vi "main.vi"() -> ()   [LabVIEW 2014]
uses:
  <vilib>/addons/Sound and Vibration/svt_Controls/subVIs/Multiplot Octave Graph.ctl
  <vilib>/Utility/NIReport.llb/NI_report.lvclass
  <vilib>/Utility/NIReport.llb/HTML Report Image Alignment.ctl
  <vilib>/sound2/lvsound2.llb/Sound File Read Open.vi
  <vilib>/sound2/lvsound2.llb/Sound File Info (refnum).vi
  <vilib>/sound2/lvsound2.llb/Sound File Read (DBL).vi
  <vilib>/addons/Sound and Vibration/svt_Octave/SVT Third-octave Analysis (1 Ch).vi
  <vilib>/addons/Sound and Vibration/svt_Octave/SVT Octave Analysis (1 Ch).vi
  <vilib>/measure/matone.llb/Harmonic Distortion Analyzer 1 Chan.vi
  <vilib>/addons/Sound and Vibration/svt_Transients/SVT STFT vs Time (Intensity).vi
  <vilib>/printing/ReportDocExtensions.llb/Append Front Panel Image to Report (path).vi
  <vilib>/addons/Sound and Vibration/svt_Octave/SoundVib_Octave.lvlib
  <vilib>/Analysis/NI_AALPro.lvlib
  <vilib>/measure/NI_MAPro.lvlib
  <vilib>/addons/Sound and Vibration/svt_Transients/SoundVib_Transient.lvlib
  <vilib>/Utility/NIReport.llb/Excel/NI_Excel.lvclass
  <vilib>/Utility/NIReport.llb/NI_ReportGenerationCore.lvlib
panel:
  in  "Print Button":bool
  in  "Help Button":bool
  in  "Tab Control":T1(tab)
  out "Wave":dbl[][](graph)
  in  "Play":bool
  in  "Pa / dBA":bool
  out "Multiplot":T2
  in  "Octave":bool
  in  "Тип анализа":u16(ring)=1 items=["1/3 октавный", "Октавный"]
  in  "Режим усреднения":u16(ring)=1 items=["Linear", "Exponential", "Equal confidence", "Peak"]
  out "Эталон":T3 {"band power" format="%#.2g"}
  out "Разность":T3 {"band power" format="%#.2g"}
  out "FFT 2":dbl[][](graph)
  out "Ампл. спектр (от. ед.)":dbl[][](array[numeric])
  out "THD (%)":dbl[](array[numeric])
  in  "FFT":bool
  in  "Режим экспорта THD":T4(ring)
  out "STFT":dbl[][](graph)
  in  "SFFT":bool
  in  "Тип оконной обработки":T5(ring)=enum."Hanning"
  in  "Время анализа (%)":dbl=50.0 min=1.0 max=100.0 step=1.0
  in  "Тип отображения":T6(ring)=enum."rainbow"
  out "Selected":i32
  in  "Обрабатываемый файл":string(combo)
  out "Start":i32
  out "Finish":i32
  in  "Clear":bool
  in  "stop":bool
  in  "TypeD":T7=enum."Open Files"
  in  "Open Files":bool
  # "Автоматизированная система объективизации оценки степени совпадения двух сравниваемых электронных звуковых рядов по заданому набору параметров"
  # "Осн. частота (Гц)"
  # "Мощность (дБ)"
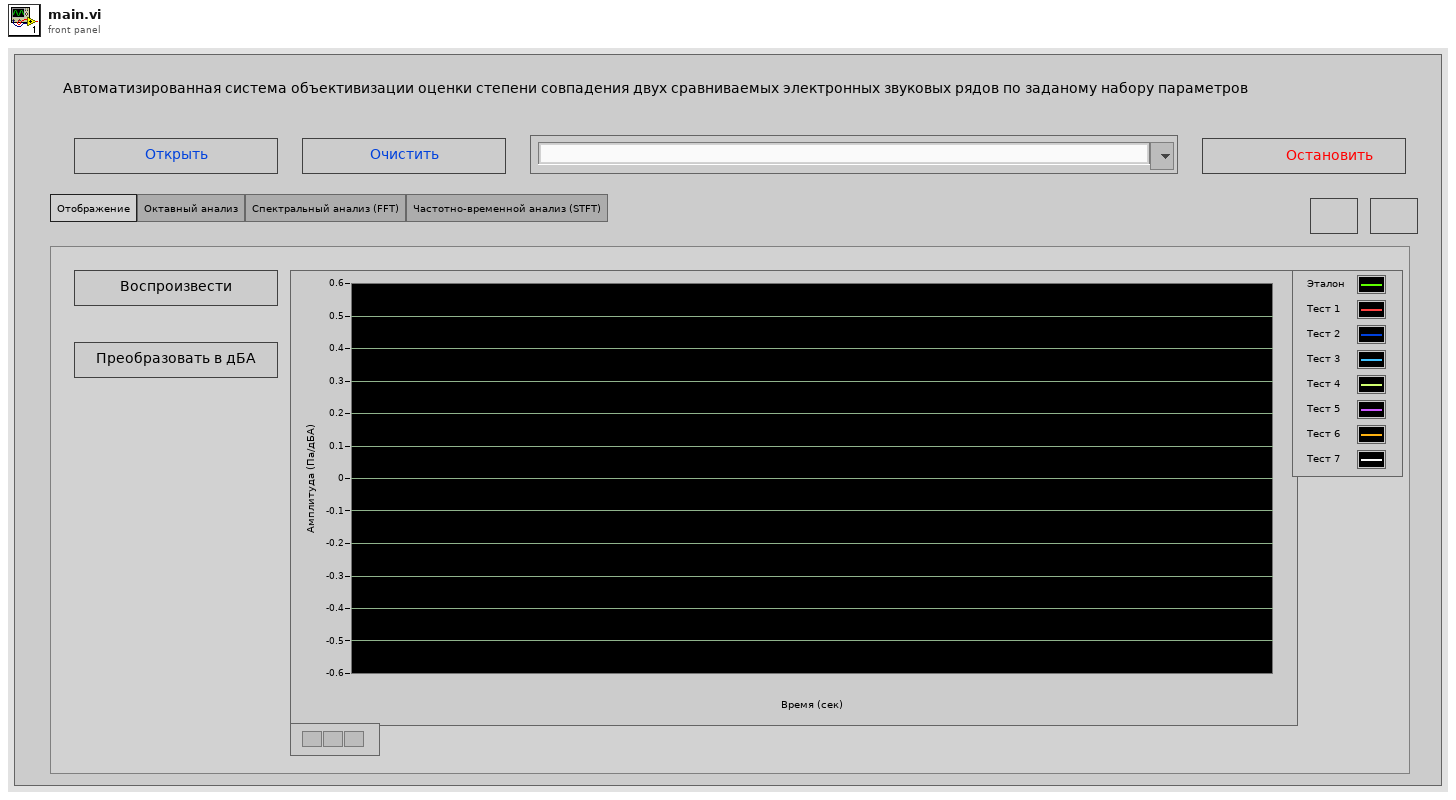
[diagram p1: front panel]
types:
  T1 = enum32{"Отображение", "Октавный анализ", "Спектральный анализ (FFT)", "Частотно-временной анализ (STFT)"}
  T2 = typedef "Multiplot Octave Graph.ctl" = cluster{"nominal frequencies [Hz]":dbl[], "band power [dB EU]":dbl[]}[]
  T3 = cluster{"nominal frequencies [Hz]":dbl[], "band power":dbl[]}
  T4 = enum16{"none", "input signal", "fundamental signal", "residual signal", "harmonics only", "noise and spurs"}
  T5 = enum16{"None ", "Hanning", "Hamming", "Blackman-Harris", "Exact Blackman", "Blackman", "Flat Top", "4 Term B-Harris ", "7 Term B-Harris", "Low Sidelobe"}
  T6 = enum16{"fire", "rainbow", "grey", "inverse grey", "ice", "original"}
  T7 = typedef "TypeDef1.ctl" = enum16{"Initialize", "Idle", "Open Files", "Pa_dBA", "FFT", "SFFT", "Play", "Octave", "Print", "Shutdown"}
  T8 = cluster{"nominal frequencies [Hz]":dbl[], "band power":dbl[]}[]
  T9 = enum16{"open", "open or create", "create or replace", "create", "open (read only)"}
  T10 = cluster{" mode":enum16{"Slow", "Fast", "Impulse", "Custom"}, "time constant [ms]":dbl}
  T11 = cluster{"low band":enum16{"20 Hz", "25 Hz", "31.5 Hz", "40 Hz", "50 Hz", "63 Hz", "80 Hz", "100 Hz", "125 Hz", "160 Hz", "200 Hz", "250 Hz", "315 Hz", "400 Hz", "500 Hz", "630 Hz", "800 Hz", "1000 Hz", "1250 Hz", "1600 Hz", "2000 Hz", "2500 Hz", "3150 Hz", "4000 Hz", "5000 Hz", "6300 Hz", "8000 Hz", "10000 Hz", "12500 Hz", "16000 Hz", "20000 Hz"}, "high band":enum16{"20 Hz", "25 Hz", "31.5 Hz", "40 Hz", "50 Hz", "63 Hz", "80 Hz", "100 Hz", "125 Hz", "160 Hz", "200 Hz", "250 Hz", "315 Hz", "400 Hz", "500 Hz", "630 Hz", "800 Hz", "1000 Hz", "1250 Hz", "1600 Hz", "2000 Hz", "2500 Hz", "3150 Hz", "4000 Hz", "5000 Hz", "6300 Hz", "8000 Hz", "10000 Hz", "12500 Hz", "16000 Hz", "20000 Hz"}}
  T12 = cluster{"low band":enum16{"16 Hz", "31.5 Hz", "63 Hz", "125 Hz", "250 Hz", "500 Hz", "1000 Hz", "2000 Hz", "4000 Hz", "8000 Hz", "16000 Hz"}, "high band":enum16{"16 Hz", "31.5 Hz", "63 Hz", "125 Hz", "250 Hz", "500 Hz", "1000 Hz", "2000 Hz", "4000 Hz", "8000 Hz", "16000 Hz"}}
  T13 = typedef "NI_ReportGenerationCore.lvlib/HTML Report Image Alignment.ctl" = enum16{"(default)", "LEFT", "RIGHT", "TOP", "TEXTTOP", "MIDDLE", "ABSMIDDLE", "BASELINE", "BOTTOM", "ABSBOTTOM"}
  T14 = enum16{"Standard Report", "HTML", "Word", "Excel"}
  T15 = typedef "Sound File Refnum.ctl" = refnum<file>
  T16 = typedef "SoundVib_Octave.lvlib/sv_Octave Info.ctl" = cluster{"standard":enum16{"ANSI S.1.11", "IEC 1260"}, "bandwidth":enum16{"1 octave", "1/3 octave", "1/6 octave", "1/12 octave", "1/24 octave"}, "low band":i32, "high band":i32, "weighting filter":T17, "dB reference":dbl, "dB On":bool, "unit label":string, "channel name":string, "description":string, "engineering units":T18, "custom label":string, "spectrum type":enum16{"power", "magnitude"}, "spectral density":bool, "filters settled":bool}
  T17 = typedef "svc_Weighting Filter Text Ring.ctl" = u16
  T18 = typedef "svc_Engineering Units Text Ring.ctl" = u16
  T19 = cluster{dbl, dbl, "Время анализа (%)":dbl, "time increment units (%)":enum16{"%", "s", "ms"}}
  T20 = enum32{"invalid app kind", "Development System", "Run Time System", "Student Edition", "Embedded LabVIEW", "Evaluation", "Custom"}
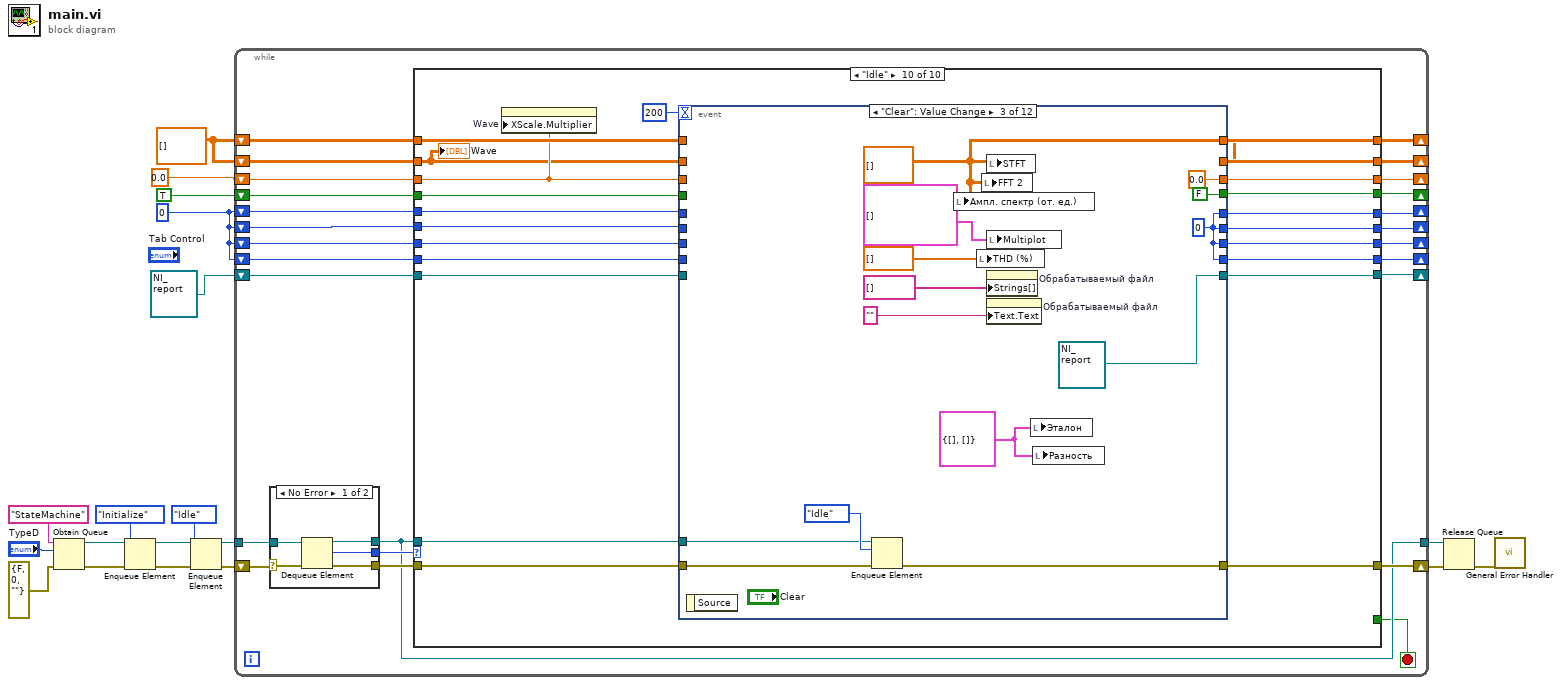
[diagram p0: block diagram]
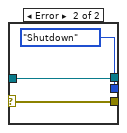
[diagram p2: hidden frame]
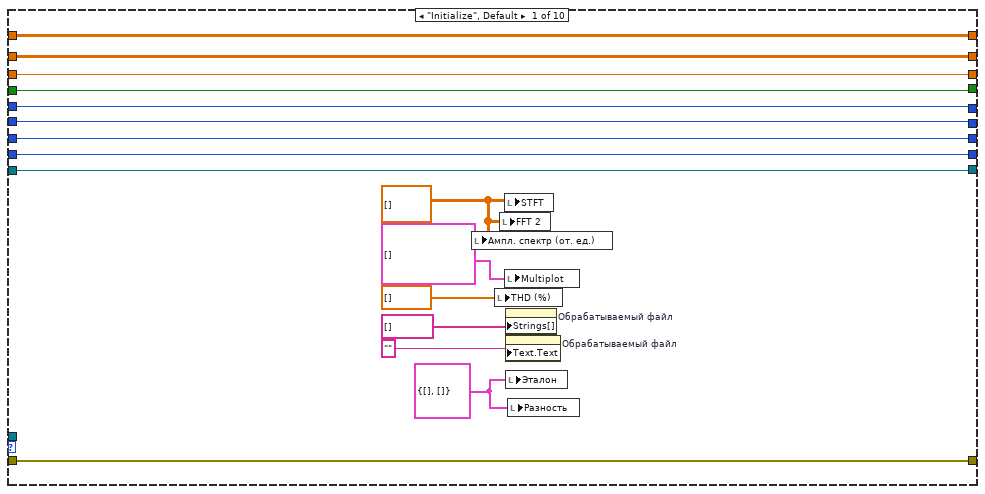
[diagram p3: hidden frame]
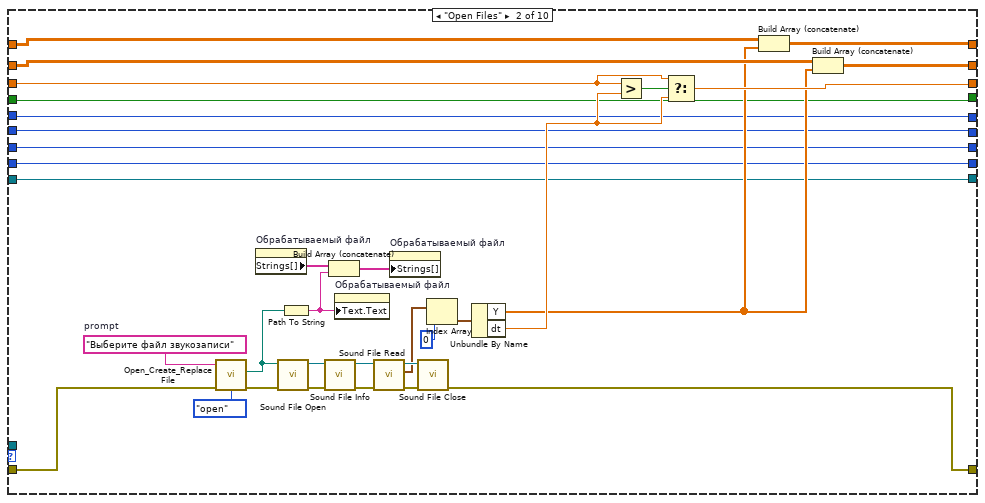
[diagram p4: hidden frame]
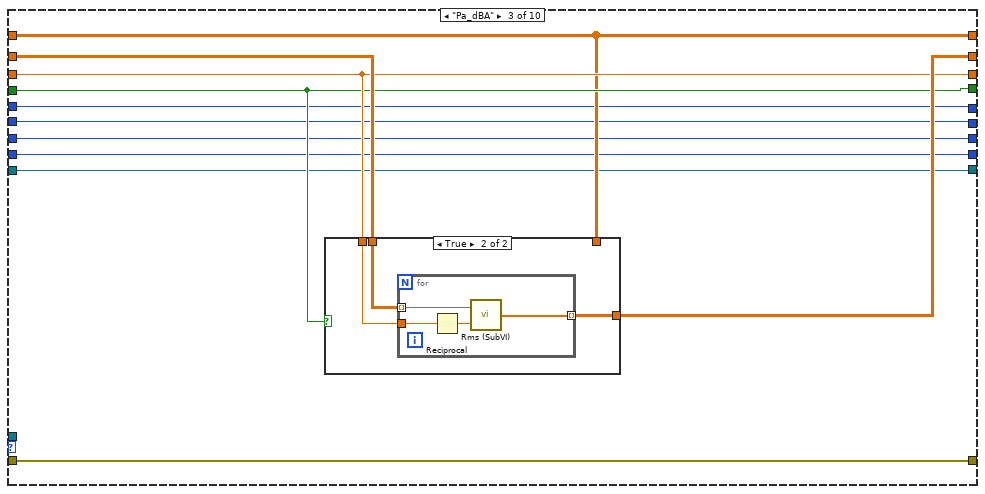
[diagram p5: hidden frame]
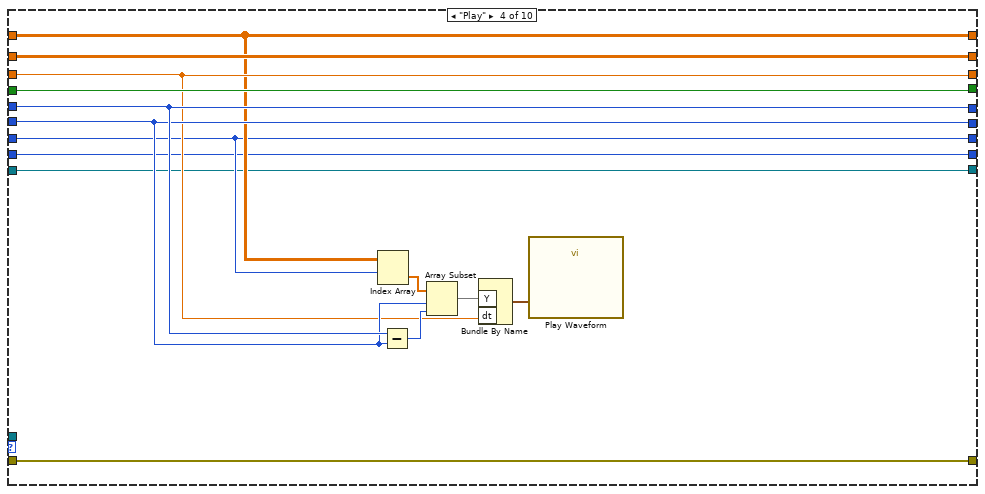
[diagram p7: hidden frame]
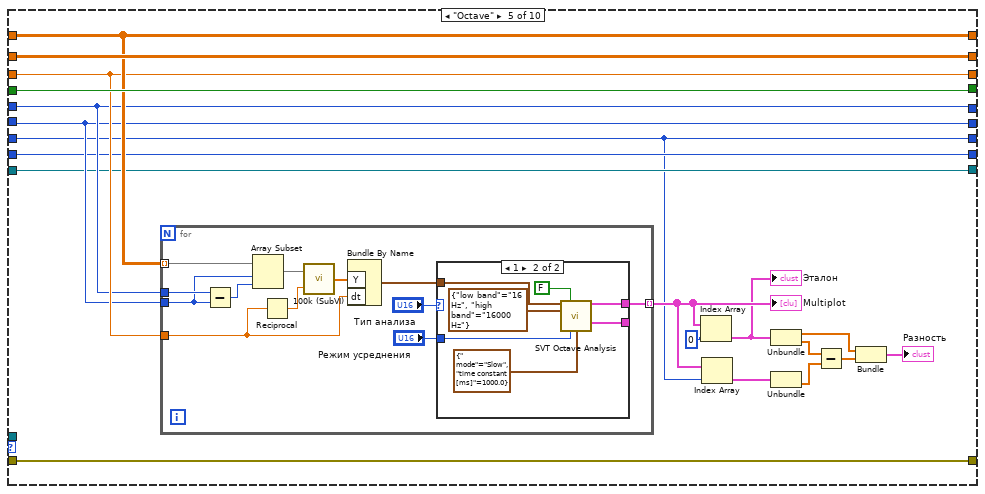
[diagram p8: hidden frame]
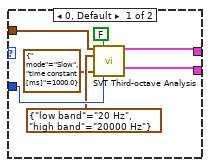
[diagram p9: hidden frame]
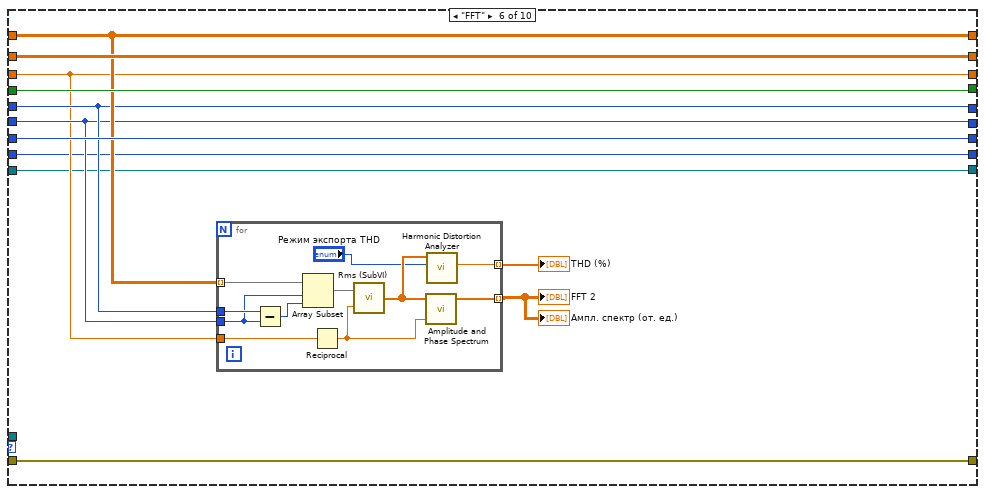
[diagram p10: hidden frame]
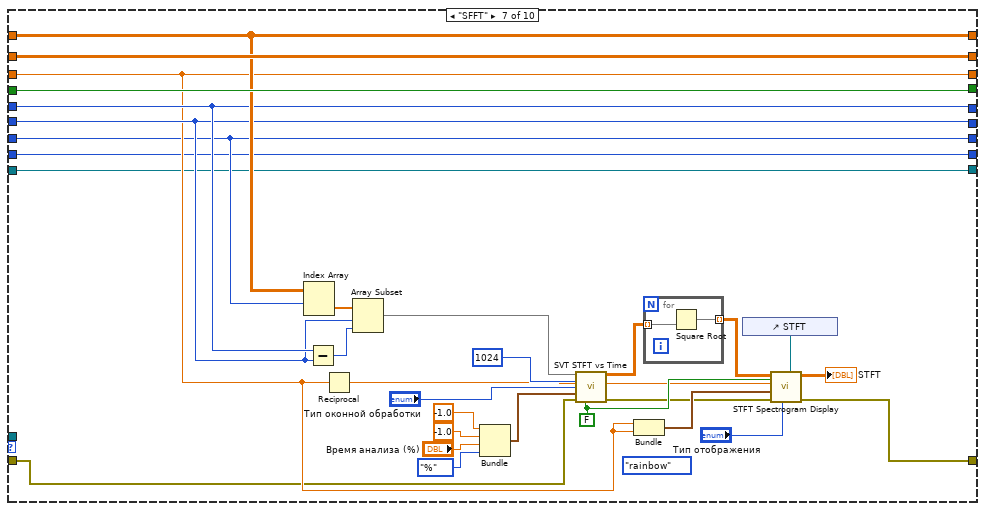
[diagram p11: hidden frame]
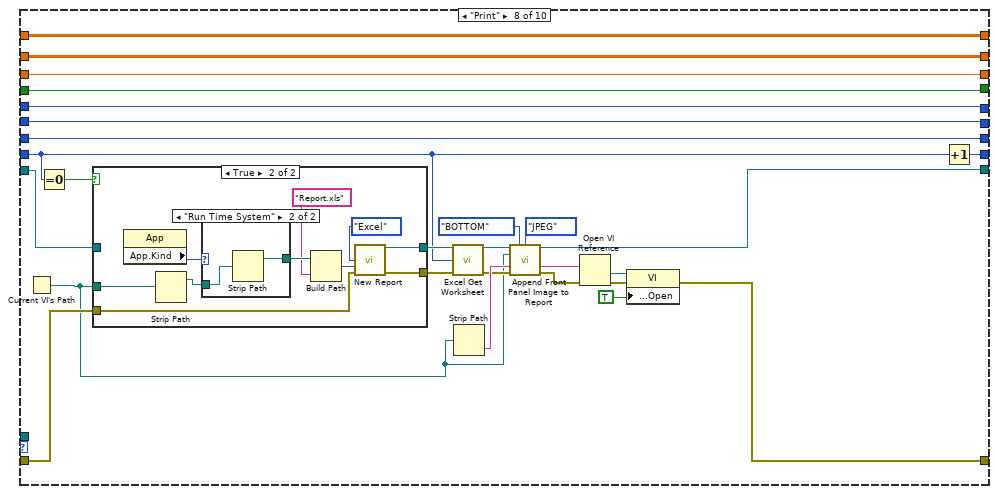
[diagram p12: hidden frame]
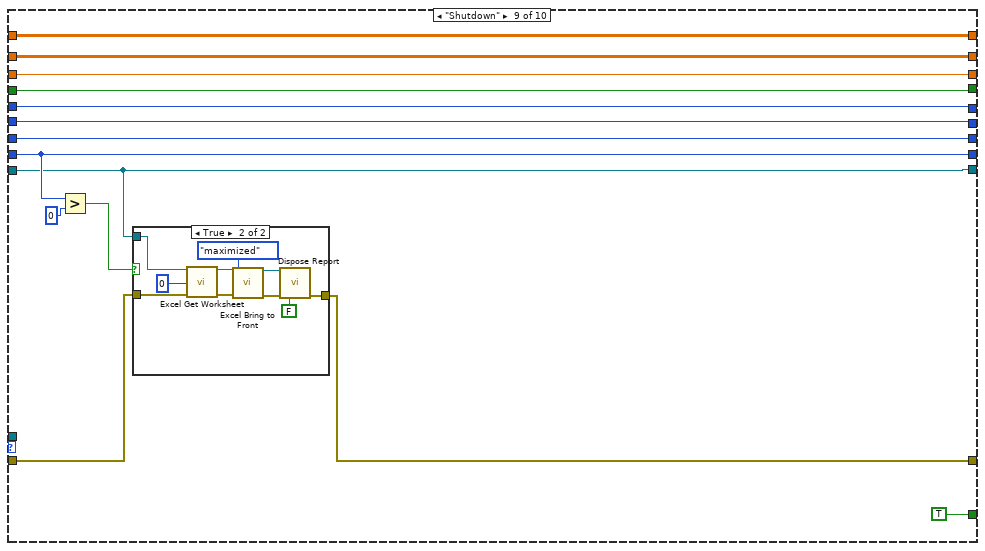
[diagram p15: hidden frame]
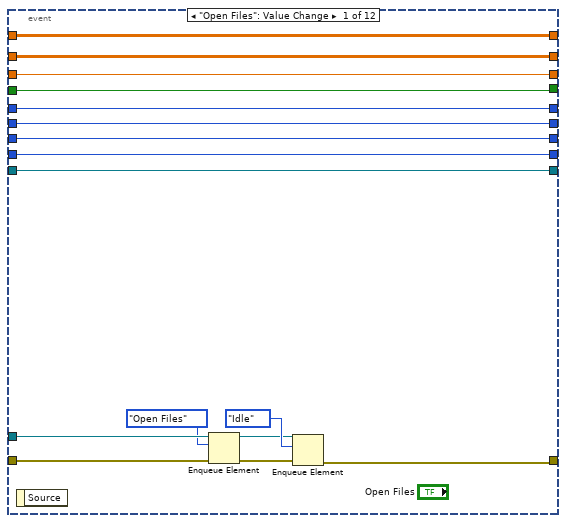
[diagram p17: hidden frame]
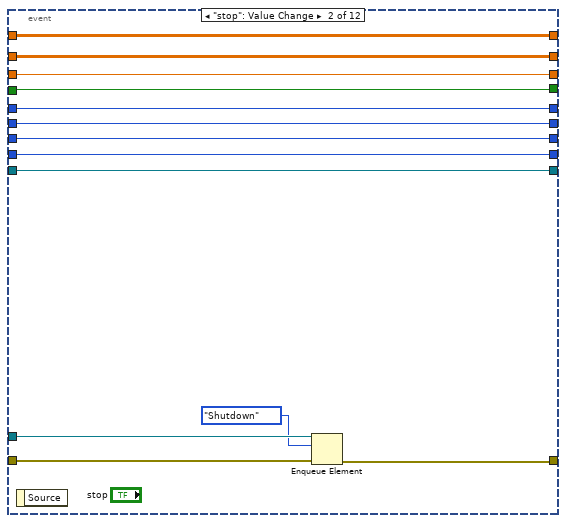
[diagram p18: hidden frame]
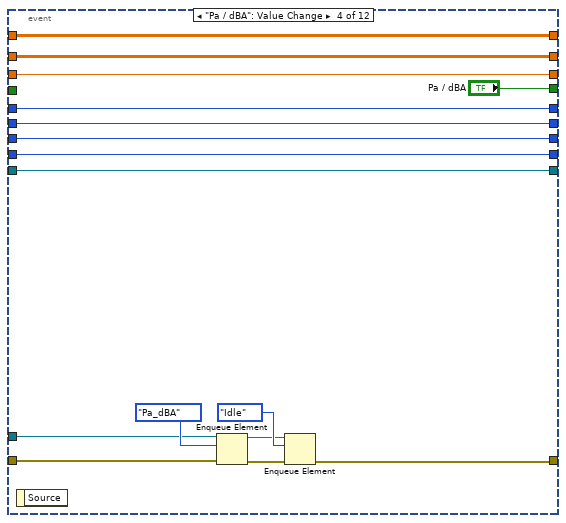
[diagram p19: hidden frame]
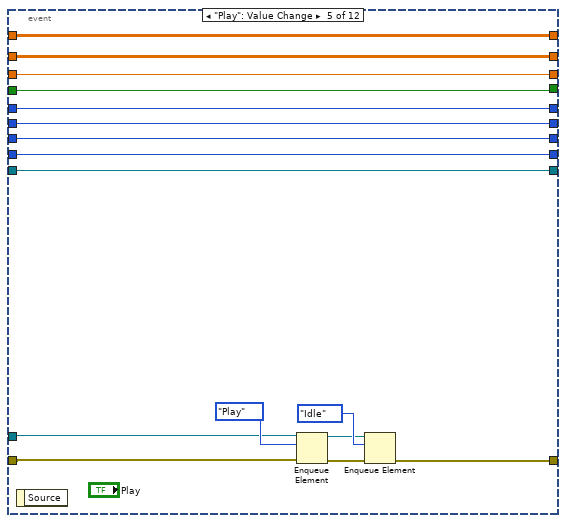
[diagram p20: hidden frame]
diagram:
  w3 = 0
  w9 = dbl[][] []
  n1 = Obtain Queue(name (unnamed)="StateMachine", element data type="TypeD", error in (no error)=errorcluster {"status"=FALSE, "code"=0, "source"=""}) -> (queue out=w19:refnum<queue>, error out=w18:errorcluster)  [unwired: 2 in, 1 out]
  n2 = Enqueue Element(queue=w19, element=TypeDef1."Initialize", error in (no error)=w18) -> (queue out=w7:refnum<queue>, error out=w6:errorcluster)  [unwired: 1 in, 1 out]
  n3 = Enqueue Element(queue=w7, element=TypeDef1."Idle", error in (no error)=w6) -> (queue out=w4:refnum<queue>, error out=w5:errorcluster)  [unwired: 1 in, 1 out]
  n4 = while {
    tunnel: w4 -> [w43]
    shift-right: [w40] -> w13
    shift-left: w5 -> [w44]
    tunnel: [w39] -> w12
    shift-right: [w36] -> _
    shift-left: w9 -> [w37]
    shift-right: [w35] -> _
    shift-left: 0.0 -> [w24]
    shift-right: [w33] -> _
    shift-left: TRUE -> [w34]
    shift-right: [w31] -> _
    shift-left: w9 -> [w32]
    shift-right: [w28] -> _
    shift-left: w3 -> [w30]
    shift-right: [w27] -> _
    shift-left: w3 -> [w29]
    shift-right: [w25] -> _
    shift-left: w3 -> [w26]
    shift-right: [w22] -> _
    shift-left: w3 -> [w23]
    shift-right: [w20] -> _
    shift-left: refnum<class "NI_report.lvclass"> refnum ("report in") -> [w21]
    stop <- w38 stop-if-true
    n5 = case shown="No Error" w44 {
      selector: w44 -> [w49 w51]
      tunnel: w43 -> [w48 w52]
      tunnel: [w47 w52] -> w39
      tunnel: [w46 w51] -> w41
      tunnel: [w45 TypeDef1."Shutdown"] -> w42
      frame No Error {
        n6 = Dequeue Element(queue=w48, error in (no error)=w49) -> (queue out=w47:refnum<queue>, element=w45:T7, error out=w46:errorcluster)  [unwired: 1 in, 1 out]
      }
      frame Error {
      }
    }
    n7 = case shown="\"Idle\"" w42 {
      tunnel: w41 -> [w68 w72 w112 w124 w151 w184 w211 w251 w278 w322]
      tunnel: [w68 w88 w112 w124 w151 w184 w215 w236 w277 w321] -> w40
      tunnel: w39 -> [_ _ _ _ _ _ _ _ _ w320]
      tunnel: [_ _ _ _ _ _ _ _ TRUE _] -> w38
      tunnel: w37 -> [w67 w89 w111 w126 w152 w191 w232 w259 w288 w310]
      tunnel: [w67 w90 w110 w126 w152 w191 w232 w259 w288 w319] -> w36
      tunnel: [w66 w84 w109 w127 w149 w185 w219 w258 w287 w318] -> w35
      tunnel: w24 -> [w66 w86 w109 w127 w149 w185 w219 w258 w287 w313]
      tunnel: w34 -> [w65 w77 w108 w130 w153 w190 w231 w257 w285 w317]
      tunnel: [w65 w77 w108 w130 w153 w190 w231 w257 w285 w316] -> w33
      tunnel: w32 -> [w64 w83 w107 w125 w150 w188 w222 w260 w286 w315]
      tunnel: [w64 w81 w107 w125 w150 w188 w222 w260 w286 w314] -> w31
      tunnel: w30 -> [w63 w80 w106 w129 w148 w187 w221 w256 w284 w307]
      tunnel: w29 -> [w62 w79 w105 w128 w147 w186 w220 w255 w283 w306]
      tunnel: [w63 w80 w106 w129 w148 w187 w221 w256 w284 w312] -> w28
      tunnel: [w62 w79 w105 w128 w147 w186 w220 w255 w283 w311] -> w27
      tunnel: w26 -> [w61 w78 w104 w123 w142 w189 w218 w254 w282 w305]
      tunnel: [w61 w78 w104 w123 w142 w189 w218 w254 w282 w308] -> w25
      tunnel: w23 -> [w55 w70 w103 w122 w146 w181 w204 w237 w281 w304]
      tunnel: [w55 w70 w103 w122 w146 w181 w204 w253 w281 w303] -> w22
      tunnel: w21 -> [w54 w69 w102 w121 w145 w180 w203 w238 w276 w302]
      tunnel: [w54 w69 w102 w121 w145 w180 w203 w235 w276 w301] -> w20
      frame "Initialize", Default {
        w53 = cluster{dbl[], dbl[]} {[], []}
        w56 = dbl[][] []
        n8 = local write "Ампл. спектр (от. ед.)"(w56) -> ()
        n9 = local write "THD (%)"(dbl[] []) -> ()
        n10 = local write "FFT 2"(w56) -> ()
        n11 = local write "STFT"(w56) -> ()
        n12 = local write "Multiplot"(T8 []) -> ()
        n13 = property on="Обрабатываемый файл" class="CmbBox"("Strings[]"=string[] []) -> ()  [unwired: 2 in, 2 out]
        n14 = property on="Обрабатываемый файл" class="CmbBox"("Text.Text"="") -> ()  [unwired: 2 in, 2 out]
        n15 = local write "Эталон"(w53) -> ()
        n16 = local write "Разность"(w53) -> ()
      }
      frame "Open Files" {
        w100 = "Выберите файл звукозаписи"  # prompt
        n17 = call <vilib>:"Open_Create_Replace File.vi"("prompt"=w100, "error in (no error)"=w72, "function (open:0)"=T9."open") -> ("error out"=w71:errorcluster, "new file path"=w76:path)  [unwired: 5 in, 2 out]
        n18 = property on="Обрабатываемый файл" class="CmbBox"() -> ("Strings[]"=w75:string[])  [unwired: 2 in, 2 out]
        n19 = call-poly <vilib>:"Sound File Open.vi"("error in (no error)"=w71, "path"=w76) -> ("error out"=w98:errorcluster, "sound file refnum"=w96:T15)  [unwired: 8 in]
        n20 = Path To String(path=w76) -> (string=w73:string)
        n21 = call-poly <vilib>:"Sound File Info.vi"("error in (no error)"=w98, "sound file refnum"=w96) -> ("error out"=w99:errorcluster, "sound file refnum out"=w97:T15)  [unwired: 6 in, 2 out]
        n22 = Build Array (concatenate)(w75, w73) -> (w74:string[])
        n23 = property on="Обрабатываемый файл" class="CmbBox"("Text.Text"=w73) -> ()  [unwired: 2 in, 2 out]
        n24 = call-poly <vilib>:"Sound File Read.vi"("error in (no error)"=w99, "sound file refnum"=w97) -> ("error out"=w94:errorcluster, "data"=w92:waveform(dbl)[], "sound file refnum out"=w95:T15)  [unwired: 5 in, 2 out]
        n25 = property on="Обрабатываемый файл" class="CmbBox"("Strings[]"=w74) -> ()  [unwired: 2 in, 2 out]
        n26 = call <vilib>:"Sound File Close.vi"("error in (no error)"=w94, "sound file refnum"=w95) -> ("error out"=w88:errorcluster)  [unwired: 9 in]
        n27 = Index Array(array=w92, index=0) -> (element=w91:waveform(dbl))
        n28 = Unbundle By Name(w91) -> ("Y"=w82:dbl[], "dt"=w85:dbl)
        n29 = Greater?(x=w86, y=w85) -> (0:w87:bool)
        n30 = Select(t=w86, s=w87, f=w85) -> (s? t:f=w84:dbl)
        n31 = Build Array (concatenate)(w83, w82) -> (w81:dbl[][])
        n32 = Build Array (concatenate)(w89, w82) -> (w90:dbl[][])
      }
      frame "Pa_dBA" {
        n33 = case shown="True" w108 {
          tunnel: w111 -> [_ w116]
          tunnel: [w113 w115] -> w110
          tunnel: w109 -> [_ w114]
          tunnel: w107 -> [w113 _]
          frame False {
          }
          frame True {
            n34 = for {
              tunnel: w116 -> [w120] mode=indexing
              tunnel: w114 -> [w117]
              tunnel: [w119] -> w115 mode=indexing
              n35 = Reciprocal(x=w117) -> (1/x=w118:dbl)
              n36 = call "Rms (SubVI).vi"("Fs"=w118, "Array"=w120) -> ("Y"=w119:dbl[])
            }
          }
        }
      }
      frame "Play" {
        n37 = Index Array(array=w125, index (row)=w123) -> (element=w131:dbl[])  [unwired: 1 in]
        n38 = Subtract(x=w129, y=w128) -> (x-y=w134:i32)
        n39 = Array Subset(array=w131, index=w128, length=w134) -> (w133:dbl[])
        n40 = Bundle By Name("Y"=w133, "dt"=w127) -> (w132:waveform(dbl))  [unwired: 1 in]
        n41 = call "Play Waveform"("Data"=w132) -> ()  [unwired: 18 in, 1 out]
      }
      frame "Octave" {
        n42 = for {
          tunnel: [w161] -> w143 mode=indexing
          tunnel: w150 -> [w160] mode=indexing
          tunnel: w149 -> [w155]
          tunnel: w148 -> [w158]
          tunnel: w147 -> [w156]
          n43 = Subtract(x=w158, y=w156) -> (x-y=w157:i32)
          n44 = Array Subset(array=w160, index=w156, length=w157) -> (w159:dbl[])
          n45 = Reciprocal(x=w155) -> (1/x=w154:dbl)
          n46 = call "100k (SubVI).vi"("Fs"=w154, "Array"=w159) -> ("Y"=w164:dbl[])
          n47 = Bundle By Name("Y"=w164, "dt"=w155) -> (w165:waveform(dbl))  [unwired: 1 in]
          n48 = case shown="1" "Тип анализа" {
            tunnel: w165 -> [w172 w179]
            tunnel: "Режим усреднения" -> [w171 w177]
            tunnel: [w169 w176] -> w161
            tunnel: [w168 w175] -> _
            frame 0, Default {
              n49 = call-poly <vilib>:"SVT Third-octave Analysis.vi"("scaled signal [EU]"=w172, "restart averaging (F)"=FALSE, "frequency range"=T11 {"low band"=enum."20 Hz", "high band"=enum."20000 Hz"}, "averaging type"=w171, "exp avg settings"=T10 {" mode"=enum."Slow", "time constant [ms]"=1000.0}) -> ("octave spectrum"=w169:T3, "octave info"=w168:T16)  [unwired: 5 in, 4 out]
            }
            frame 1 {
              n50 = call-poly <vilib>:"SVT Octave Analysis.vi"("scaled signal [EU]"=w179, "restart averaging (F)"=FALSE, "frequency range"=T12 {"low band"=enum."16 Hz", "high band"=enum."16000 Hz"}, "averaging type"=w177, "exp avg settings"=T10 {" mode"=enum."Slow", "time constant [ms]"=1000.0}) -> ("octave spectrum"=w176:T3, "octave info"=w175:T16)  [unwired: 5 in, 4 out]
            }
          }
        }
        "Multiplot" <- w143
        n51 = Index Array(array=w143, index=0) -> (element=w141:T3)
        "Эталон" <- w141
        n52 = Index Array(array=w143, index=w142) -> (element=w140:T3)
        n53 = Unbundle(w141) -> ("nominal frequencies [Hz]"=w136:dbl[], "band power"=w139:dbl[])
        n54 = Unbundle(w140) -> ("band power"=w138:dbl[])  [unwired: 1 out]
        n55 = Subtract(x=w139, y=w138) -> (x-y=w137:dbl[])
        n56 = Bundle("nominal frequencies [Hz]"=w136, w137) -> (→"Разность":cluster{"nominal frequencies [Hz]":dbl[], dbl[]})  [unwired: 1 in]
      }
      frame "FFT" {
        n57 = for {
          tunnel: w188 -> [w201] mode=indexing
          tunnel: w187 -> [w200]
          tunnel: w186 -> [w199]
          tunnel: w185 -> [w197]
          tunnel: [w198] -> w183 mode=indexing
          tunnel: [w194] -> w182 mode=indexing
          n58 = Subtract(x=w200, y=w199) -> (x-y=w202:i32)
          n59 = Array Subset(array=w201, index=w199, length=w202) -> (w195:dbl[])
          n60 = Reciprocal(x=w197) -> (1/x=w196:dbl)
          n61 = call "Rms (SubVI).vi"("Fs"=w196, "Array"=w195) -> ("Y"=w193:dbl[])
          n62 = call <vilib>:"Amplitude and Phase Spectrum.vi"("dt"=w196, "Signal (V)"=w193) -> ("Amp Spectrum Mag (Vrms)"=w198:dbl[])  [unwired: 1 in, 2 out]
          n63 = call-poly <vilib>:"Harmonic Distortion Analyzer.vi"("export mode"="Режим экспорта THD", "signal in"=w193) -> ("THD"=w194:dbl)  [unwired: 4 in, 5 out]
        }
        "FFT 2" <- w183
        "Ампл. спектр (от. ед.)" <- w183
        "THD (%)" <- w182
      }
      frame "SFFT" {
        (unwired) T6."rainbow" ("map selector")
        w226 = FALSE ("dB On (T)")
        n64 = Index Array(array=w222, index (row)=w218) -> (element=w223:dbl[])  [unwired: 1 in]
        n65 = Subtract(x=w221, y=w220) -> (x-y=w224:i32)
        n66 = Reciprocal(x=w219) -> (1/x=w214:dbl)
        n67 = Array Subset(array=w223, index=w220, length=w224) -> (w213:dbl[])
        n68 = Bundle(-1.0, -1.0, "Время анализа (%)"="Время анализа (%)", "time increment units (%)"=enum16{"%", "s", "ms"}."%") -> (w206:T19)  [unwired: 1 in]
        n69 = call-poly <vilib>:"SVT STFT vs Time.vi"("scaled signal [EU]"=w213, "FFT block size"=1024, "window"="Тип оконной обработки", "time segment"=w206, "error in (no error)"=w211, "dB On (T)"=w226) -> ("power spectra [dB EU]"=w229:dbl[][], "error out"=w216:errorcluster)  [unwired: 4 in, 4 out]
        n70 = Bundle(w219, w219) -> (w225:cluster{dbl, dbl})  [unwired: 1 in]
        n71 = for {
          tunnel: w229 -> [w233] mode=indexing
          tunnel: [w234] -> w230 mode=indexing
          n72 = Square Root(x=w233) -> (sqrt(x)=w234:dbl[])
        }
        n73 = control-ref of="STFT"() -> (w227:refnum<vi>)
        n74 = call "STFT Spectrogram Display.vi"("Intensity Graph"=w227, "map selector"="Тип отображения", "dB On"=w226, "error in (no error)"=w216, "time-freq sampling info"=w225, "dt"=w214, "STFT Spectrogram In"=w230) -> ("error out"=w215:errorcluster, "STFT Spectrogram Out"=→"STFT":dbl[][])  [unwired: 3 out]
      }
      frame "Print" {
        n75 = Current VI's Path() -> (path=w239:path)
        n76 = Equal To 0?(x=w237) -> (x = 0?=w252:bool)
        n77 = case shown="True" w252 {
          tunnel: [w262 w266] -> w240
          tunnel: w251 -> [w261 w265]
          tunnel: [w261 w264] -> w241
          tunnel: w239 -> [_ w263]
          tunnel: w238 -> [w262 _]
          frame False {
          }
          frame True {
            n78 = property class="App"() -> ("App.Kind"=w271:T20)  [unwired: 2 in, 2 out]
            n79 = Strip Path(path=w263) -> (stripped path=w269:path)  [unwired: 1 out]
            n80 = case shown="\"Run Time System\"" w271 {
              tunnel: w269 -> [w273 w275]
              tunnel: [w273 w274] -> w268
              frame Default {
              }
              frame "Run Time System" {
                n81 = Strip Path(path=w275) -> (stripped path=w274:path)  [unwired: 1 out]
              }
            }
            n82 = Build Path(base path=w268, name or relative path="Report.xls") -> (appended path=w270:path)
            n83 = call <vilib>:"New Report.vi"("report type"=T14."Excel", "template (empty)"=w270, "error in (no error)"=w265) -> ("report out"=w266:refnum<class "NI_report.lvclass">, "error out"=w264:errorcluster)  [unwired: 11 in]
          }
        }
        n84 = call <vilib>:"Excel Get Worksheet.vi"("report in"=w240, "worksheet index (0)"=w237, "error in (no error)"=w241) -> ("report out"=w249:refnum<class "NI_report.lvclass">, "error out"=w248:errorcluster)  [unwired: 11 in]
        n85 = Strip Path(path=w239) -> (name=w250:string)  [unwired: 1 out]
        n86 = call-poly <vilib>:"Append Front Panel Image to Report.vi"("report in"=w249, "alignment (default)"=HTML_Report_Image_Alignment."BOTTOM", "image format (jpeg)"=enum32{"PNG", "JPEG", "GIF"}."JPEG" ("Image Format (jpeg)"), "VI"=w239, "description"=w250, "error in (no error)"=w248) -> ("report out"=w235:refnum<class "NI_report.lvclass">, "error out"=w243:errorcluster)  [unwired: 5 in, 3 out]
        n87 = Open VI Reference(vi path=w250, error in (no error)=w243) -> (vi reference=w244:refnum<vi>, error out=w245:errorcluster)  [unwired: 4 in]
        n88 = property class="VI"(reference=w244, error in=w245, "Front Panel Window:Open"=TRUE) -> (error out=w236:errorcluster)  [unwired: 1 out]
        n89 = Increment(x=w237) -> (x+1=w253:i32)
      }
      frame "Shutdown" {
        n90 = Greater?(x=w281, y=0) -> (0:w279:bool)
        n91 = case shown="True" w279 {
          tunnel: w276 -> [_ w293]
          tunnel: w278 -> [w290 w292]
          tunnel: [w290 w299] -> w277
          frame False {
          }
          frame True {
            n92 = call <vilib>:"Excel Get Worksheet.vi"("report in"=w293, "worksheet index (0)"=0, "error in (no error)"=w292) -> ("report out"=w294:refnum<class "NI_report.lvclass">, "error out"=w295:errorcluster)  [unwired: 11 in]
            n93 = call <vilib>:"Excel Bring to Front.vi"("report in"=w294, "window state (maximized)"=enum16{"maximized", "minimized", "normal"}."maximized", "error in (no error)"=w295) -> ("report out"=w296:refnum<class "NI_report.lvclass">, "error out"=w297:errorcluster)  [unwired: 11 in]
            n94 = call-dynamic "Dispose Report.vi"("report in"=w296, "error in (no error)"=w297, "close report? (T)"=FALSE ("Close Report? (T)")) -> ("error out"=w299:errorcluster)  [unwired: 12 in]
          }
        }
      }
      frame "Idle" {
        n95 = property on="Wave" class="WFGraph (strict)"("XScale.Multiplier"=w313) -> ()  [unwired: 2 in, 2 out]
        n96 = event shown="[2] \"Clear\": Value Change" {
          selector: _ -> [_ _ _ _ _ _ _ _ _ _ _ _]
          dyn-events: _ -> [_ _ _ _ _ _ _ _ _ _ _ _]
          timeout: 200 -> [_ _ _ _ _ _ _ _ _ _ _ _]
          tunnel: w322 -> [w337 w351 w364 w380 w393 w409 w430 w448 w464 w480 w496 w503]
          tunnel: [w330 w350 w362 w375 w391 w408 w429 w446 w463 w478 w494 w501] -> w321
          tunnel: w320 -> [w338 w349 w363 w379 w392 w410 w428 w447 w465 w479 w495 w502]
          tunnel: w310 -> [w334 w346 _ w373 w386 w405 w422 w444 w456 w476 w492 w509]
          tunnel: [w334 w346 w355 w373 w386 w405 w422 w444 w456 w476 w492 w509] -> w319
          tunnel: [w335 w345 0.0 w374 w388 w406 w423 w439 w457 w475 w491 w510] -> w318
          tunnel: w313 -> [w335 w345 _ w374 w388 w406 w423 w439 w457 w475 w491 w510]
          tunnel: w317 -> [w325 w344 _ _ w387 w407 w424 w443 w458 w474 w490 w511]
          tunnel: [w325 w344 FALSE "Pa / dBA" w387 w407 w424 w443 w458 w474 w490 w511] -> w316
          tunnel: w315 -> [w329 w347 _ w371 w385 w404 w421 w445 w455 w477 w493 w508]
          tunnel: [w329 w347 w355 w371 w385 w404 w421 w445 w455 w477 w493 w508] -> w314
          tunnel: [w328 w343 w354 w370 w389 w413 w425 w442 w459 w473 w489 w512] -> w312
          tunnel: w307 -> [w328 w343 _ w370 w389 _ w425 w442 w459 w473 w489 w512]
          tunnel: w306 -> [w327 w342 _ w369 w390 _ w427 w441 w460 w472 w488 w513]
          tunnel: [w327 w342 w354 w369 w390 w412 w427 w441 w460 w472 w488 w513] -> w311
          tunnel: [w326 w341 w354 w368 w384 w401 w426 w440 w461 w471 w487 w514] -> w308
          tunnel: w305 -> [w326 w341 _ w368 w384 _ w426 w440 w461 w471 w487 w514]
          tunnel: [w324 w340 w354 w367 w383 w399 w420 w438 w454 w470 w486 w500] -> w303
          tunnel: w304 -> [w324 w340 _ w367 w383 w399 w420 w438 w454 w470 w486 w500]
          tunnel: w302 -> [w323 w339 _ w366 w382 w398 w419 w437 w453 w469 w485 w499]
          tunnel: [w323 w339 refnum<class "NI_report.lvclass"> refnum ("report in") w366 w382 w398 w419 w437 w453 w469 w485 w499] -> w301
          event "Open Files": Value Change {
            n97 = event-data() -> ()  [unwired: 1 in, 1 out]
            n98 = Enqueue Element(queue=w338, element=TypeDef1."Open Files", error in (no error)=w337) -> (queue out=w331:refnum<queue>, error out=w332:errorcluster)  [unwired: 1 in, 1 out]
            n99 = Enqueue Element(queue=w331, element=TypeDef1."Idle", error in (no error)=w332) -> (error out=w330:errorcluster)  [unwired: 1 in, 2 out]
          }
          event "stop": Value Change {
            n100 = event-data() -> ()  [unwired: 1 in, 1 out]
            n101 = Enqueue Element(queue=w349, element=TypeDef1."Shutdown", error in (no error)=w351) -> (error out=w350:errorcluster)  [unwired: 1 in, 2 out]
          }
          event "Clear": Value Change {
            w352 = cluster{dbl[], dbl[]} {[], []}
            w354 = 0
            w355 = dbl[][] []
            n102 = event-data() -> ()  [unwired: 1 in, 1 out]
            n103 = Enqueue Element(queue=w363, element=TypeDef1."Idle", error in (no error)=w364) -> (error out=w362:errorcluster)  [unwired: 1 in, 2 out]
            n104 = local write "Ампл. спектр (от. ед.)"(w355) -> ()
            n105 = local write "THD (%)"(dbl[] []) -> ()
            n106 = local write "FFT 2"(w355) -> ()
            n107 = local write "STFT"(w355) -> ()
            n108 = local write "Multiplot"(T8 []) -> ()
            n109 = property on="Обрабатываемый файл" class="CmbBox"("Strings[]"=string[] []) -> ()  [unwired: 2 in, 2 out]
            n110 = property on="Обрабатываемый файл" class="CmbBox"("Text.Text"="") -> ()  [unwired: 2 in, 2 out]
            n111 = local write "Эталон"(w352) -> ()
            n112 = local write "Разность"(w352) -> ()
          }
          event "Pa / dBA": Value Change {
            n113 = event-data() -> ()  [unwired: 1 in, 1 out]
            n114 = Enqueue Element(queue=w379, element=TypeDef1."Pa_dBA", error in (no error)=w380) -> (queue out=w377:refnum<queue>, error out=w376:errorcluster)  [unwired: 1 in, 1 out]
            n115 = Enqueue Element(queue=w377, element=TypeDef1."Idle", error in (no error)=w376) -> (error out=w375:errorcluster)  [unwired: 1 in, 2 out]
          }
          event "Play": Value Change {
            n116 = event-data() -> ()  [unwired: 1 in, 1 out]
            n117 = Enqueue Element(queue=w392, element=TypeDef1."Play", error in (no error)=w393) -> (queue out=w395:refnum<queue>, error out=w394:errorcluster)  [unwired: 1 in, 1 out]
            n118 = Enqueue Element(queue=w395, element=TypeDef1."Idle", error in (no error)=w394) -> (error out=w391:errorcluster)  [unwired: 1 in, 2 out]
          }
          event Timeout {
            n119 = event-data() -> ()  [unwired: 1 in, 1 out]
            n120 = Reciprocal(x=w406) -> (1/x=w418:dbl)
            n121 = property on="Обрабатываемый файл" class="CmbBox"() -> ("Strings[]"=w403:string[], "Value"=w402:string)  [unwired: 2 in, 2 out]
            n122 = property on="Wave" class="WFGraph (strict)"() -> ("XScale.Maximum"=w414:dbl)  [unwired: 2 in, 2 out]
            n123 = property on="Wave" class="WFGraph (strict)"() -> ("XScale.Minimum"=w415:dbl)  [unwired: 2 in, 2 out]
            n124 = Enqueue Element(queue=w410, element=TypeDef1."Idle", error in (no error)=w409) -> (error out=w408:errorcluster)  [unwired: 1 in, 2 out]
            n125 = Search 1D Array(1D array=w403, element=w402) -> (index of element=w401:i32)  [unwired: 1 in]
            n126 = Multiply(x=w418, y=w415) -> (x*y=w417:dbl)
            n127 = Multiply(x=w414, y=w418) -> (x*y=w416:dbl)
            n128 = Increment(x=w401) -> (x+1=→"Selected":i32)
            n129 = To Long Integer(number=w417) -> (32bit integer=w412:i32)
            "Start" <- w412
            n130 = To Long Integer(number=w416) -> (32bit integer=w413:i32)
            "Finish" <- w413
          }
          event Panel Close? {
            n131 = event-data() -> ()  [unwired: 1 in, 1 out]
            n132 = Enqueue Element(queue=w428, element=TypeDef1."Idle", error in (no error)=w430) -> (error out=w429:errorcluster)  [unwired: 1 in, 2 out]
            n133 = Two Button Dialog(message="Завершить работу с потерей всех\nнесохраненных данных? ", 1:"Нет" ("F button name (\"Cancel\")"), 2:"Да" ("T button name (\"OK\")")) -> (T button?=w436:bool)
            n134 = Not(x=w436) -> (.not. x?=w432:bool)
            n135 = event-data("Discard?"=w432) -> ()  [unwired: 1 in, 1 out]
          }
          event "Octave": Value Change {
            n136 = event-data() -> ()  [unwired: 1 in, 1 out]
            n137 = Enqueue Element(queue=w447, element=TypeDef1."Octave", error in (no error)=w448) -> (queue out=w450:refnum<queue>, error out=w449:errorcluster)  [unwired: 1 in, 1 out]
            n138 = Enqueue Element(queue=w450, element=TypeDef1."Idle", error in (no error)=w449) -> (error out=w446:errorcluster)  [unwired: 1 in, 2 out]
          }
          event "FFT": Value Change {
            n139 = event-data() -> ()  [unwired: 1 in, 1 out]
            n140 = Enqueue Element(queue=w465, element=TypeDef1."FFT", error in (no error)=w464) -> (queue out=w467:refnum<queue>, error out=w466:errorcluster)  [unwired: 1 in, 1 out]
            n141 = Enqueue Element(queue=w467, element=TypeDef1."Idle", error in (no error)=w466) -> (error out=w463:errorcluster)  [unwired: 1 in, 2 out]
          }
          event "SFFT": Value Change {
            n142 = event-data() -> ()  [unwired: 1 in, 1 out]
            n143 = Enqueue Element(queue=w479, element=TypeDef1."SFFT", error in (no error)=w480) -> (queue out=w483:refnum<queue>, error out=w484:errorcluster)  [unwired: 1 in, 1 out]
            n144 = Enqueue Element(queue=w483, element=TypeDef1."Idle", error in (no error)=w484) -> (error out=w478:errorcluster)  [unwired: 1 in, 2 out]
          }
          event "Help Button": Value Change {
            n145 = event-data() -> ()  [unwired: 1 in, 1 out]
            n146 = Enqueue Element(queue=w495, element=TypeDef1."Idle", error in (no error)=w496) -> (error out=w494:errorcluster)  [unwired: 1 in, 2 out]
            n147 = Control Help Window(1:TRUE ("Show")) -> ()  [unwired: 1 in]
          }
          event "Print Button": Value Change {
            n148 = event-data() -> ()  [unwired: 1 in, 1 out]
            n149 = Enqueue Element(queue=w502, element=TypeDef1."Print", error in (no error)=w503) -> (queue out=w506:refnum<queue>, error out=w507:errorcluster)  [unwired: 1 in, 1 out]
            n150 = Enqueue Element(queue=w506, element=TypeDef1."Idle", error in (no error)=w507) -> (error out=w501:errorcluster)  [unwired: 1 in, 2 out]
          }
        }
        "Wave" <- w310
      }
    }
  }
  n151 = Release Queue(queue=w12, error in (no error)=w13) -> (error out=w2:errorcluster)  [unwired: 1 in, 2 out]
  n152 = call <vilib>:"General Error Handler.vi"("error in (no error)"=w2) -> ()  [unwired: 10 in, 5 out]
